vi "Get Local Lookup.vi"(8 "error in (no error)":errorcluster, 11 "Process in":refnum<class "Process.lvclass">) -> (0 "error out":errorcluster, 2 "Process Lookup":T1, 3 "Process out":refnum<class "Process.lvclass">)   [LabVIEW 2019, in "TimingDRV Engine.lvlib" / "Process.lvclass"]
uses:
  Process.lvclass
  TypeDefs/Process Lookup.ctl
  TypeDefs/Message.ctl
  TypeDefs/Update.ctl
  Process.lvclass/Process.ctl
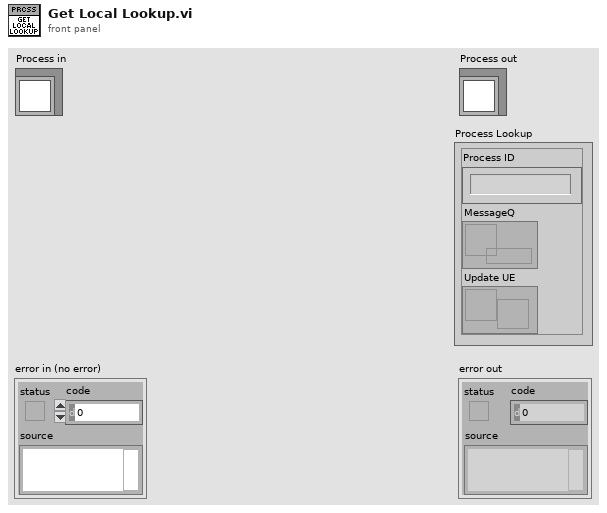
[diagram p1: front panel]
types:
  T1 = typedef "TimingDRV Engine.lvlib/Process.lvclass/Process Lookup.ctl" = cluster{"Process ID":string, "MessageQ":refnum<queue>, "Update UE":refnum<user-event>}
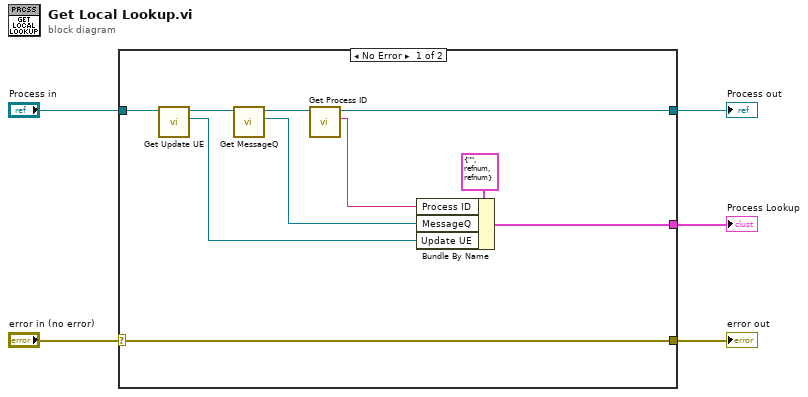
[diagram p0: block diagram]
diagram:
  n1 = case shown="No Error" "error in (no error)" {
    selector: "error in (no error)" -> [w15 w17]
    tunnel: [w15 w17] -> w4
    tunnel: [w10 w16] -> w2
    tunnel: "Process in" -> [w8 w16]
    tunnel: [w9 _] -> w1
    frame No Error {
      n2 = call "Get Update UE.vi"("CD_Process in"=w8) -> ("Update UE"=w6:refnum<user-event>, "CD_Process out"=w7:refnum<class "Process.lvclass">)  [unwired: 9 in]
      n3 = call "Get MessageQ.vi"("CD_Process in"=w7) -> ("MessageQ"=w11:refnum<queue>, "CD_Process out"=w13:refnum<class "Process.lvclass">)  [unwired: 9 in]
      n4 = call "Get Process ID.vi"("CD_Process in"=w13) -> ("Process ID"=w12:string, "CD_Process out"=w10:refnum<class "Process.lvclass">)  [unwired: 9 in]
      n5 = Bundle By Name(cluster=T1 {"Process ID"="", "MessageQ"=refnum, "Update UE"=refnum} ("Process Lookup"), "Process ID"=w12, "MessageQ"=w11, "Update UE"=w6) -> (w9:T1)
    }
    frame Error {
    }
  }
  "error out" <- w4
  "Process out" <- w2
  "Process Lookup" <- w1
